vi "FPGA Main Default.vi"() -> ()   [LabVIEW 2019]
doc: "The myRIO v1.1 FPGA Shipping Personality. This personality contains support for:\n- 2 Analog Input Interrupt channel\n- 4 Digital Input Interrupt channel\n- 1 Timer\n- 1 Accelerometer\n- 1 Button\n- 4 LED\n- 10 Analog Input channels with 1 Sample\n- 6 Analog Output channels with 1 Sample\n- 40 Digital I/O channels with 1 Sample\n- 2 I2C channels\n- 4 Encoder channels\n- 6 PWM channels\n- 2 SPI channels"
uses:
  <vilib>/rvi/Emulation/niFpgaGetClockAttributes.vi
  <vilib>/rvi/Emulation/niFpgaSctlEmulationGetInTimedLoop.vi
  <vilib>/rvi/Emulation/niFpgaEmulationReportErrorSimple.vi
  <vilib>/rvi/Emulation/niFpgaProcessEmulError.vi
  <vilib>/rvi/eio/common/nirviEmuTemplateMethod_errors.vi
  <vilib>/rvi/Emulation/niFpgaCriticalErrorInLSC.vi
  <vilib>/eio/EIONode/EIONode.xnode
panel:
  in  "Synchronization":bool
  in  "OutputPinMap":u8
  out "PinMap":bool[](array[boolean])
  out "DIO_indicator":bool[](array[boolean])
  out "Camera_triggerin":bool
  out "Camera_triggerout":bool
  in  "PulseNumberperLoop":i32
  in  "Trigger":u64
  in  "BreakinLoop":bool
  in  "OFFTime":u32
  in  "ONTime":u32
  # "Camera trigger port: A:DIO8\nLight source port: B:DIO1~7, 1~6 are Normally Open (NO), 7 is  NC."
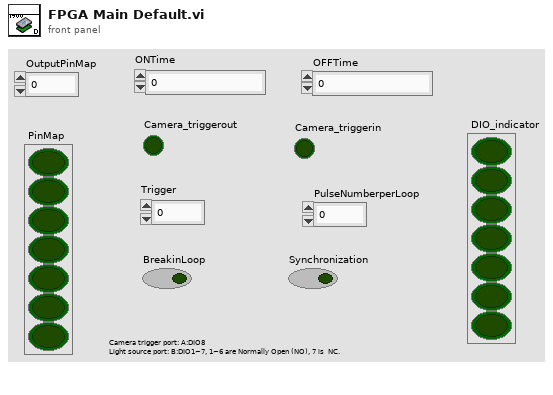
[diagram p1: front panel]
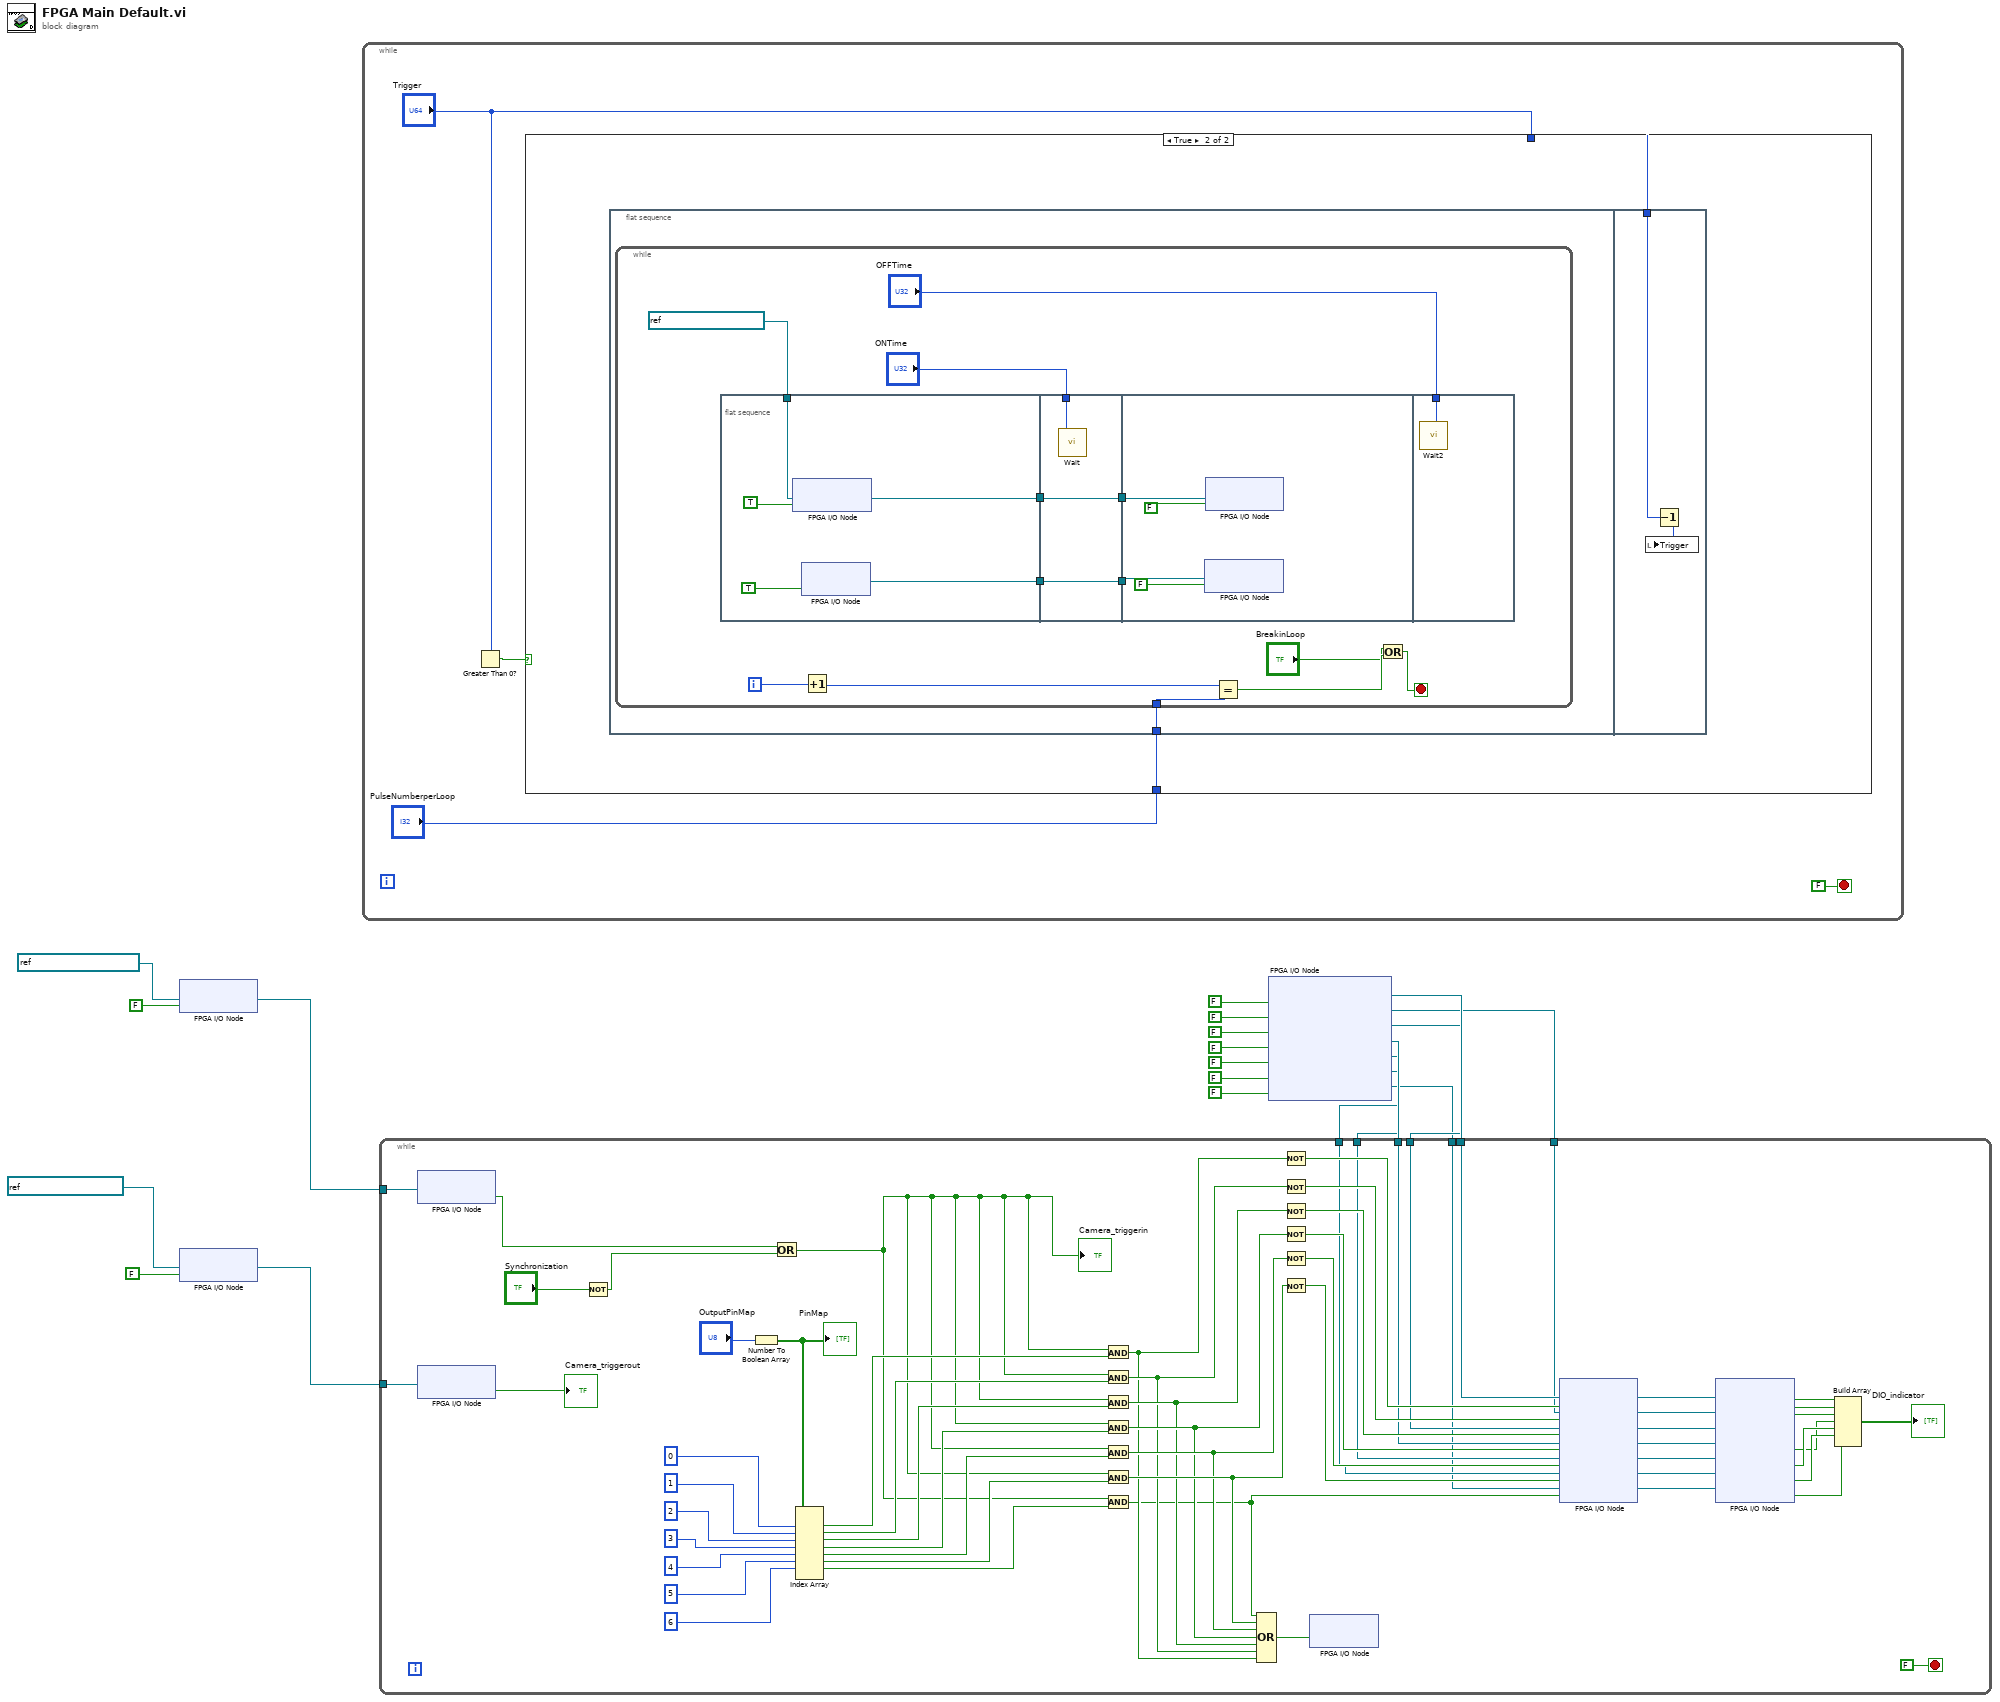
[diagram p0: block diagram]
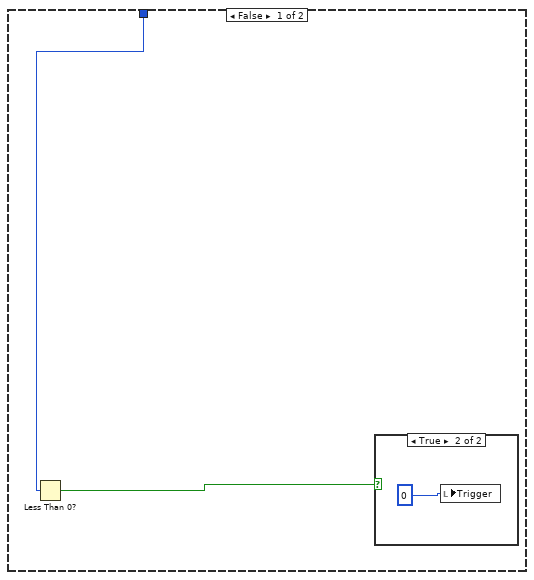
[diagram p2: hidden frame]
diagram:
  n1 = xnode "FPGA I/O Node"("I/O Item"=FALSE ("ConnectorB/DIO7"), "FPGA I/O In"=refnum<k21> "ConnectorA/DIO15") -> ("FPGA I/O Out"=w14:refnum<k21>)
  n2 = xnode "FPGA I/O Node"("I/O Item"=FALSE ("ConnectorA/DIO8"), "FPGA I/O In"=refnum<k21> "ConnectorA/DIO8") -> ("FPGA I/O Out"=w17:refnum<k21>)
  n3 = while {
    stop <- FALSE stop-if-true
    n4 = Greater Than 0?(x="Trigger") -> (x > 0?=w23:bool)
    n5 = case shown="True" w23 {
      tunnel: "PulseNumberperLoop" -> [_ w29]
      tunnel: "Trigger" -> [w26 w28]
      frame False {
        n6 = Less Than 0?(x=w26) -> (x < 0?=w25:bool)
        n7 = case shown="True" w25 {
          frame False {
          }
          frame True {
            n8 = local write "Trigger"(i16 0) -> ()
          }
        }
      }
      frame True {
        n9 = flat-sequence {
          tunnel: w29 -> [w30]
          tunnel: w28 -> [w57]
          frame #0 {
            n10 = while {
              tunnel: w30 -> [w38]
              i -> [w39]
              stop <- w41 stop-if-true
              n11 = flat-sequence {
                tunnel: refnum<k21> "ConnectorA/DIO8" ("FPGA I/O In") -> [w46]
                tunnel: [w45] -> w33
                tunnel: [w44] -> w31
                tunnel: "ONTime" -> [w51]
                tunnel: [w50] -> w34
                tunnel: w33 -> [w50]
                tunnel: [w49] -> w32
                tunnel: w31 -> [w49]
                tunnel: w34 -> [w53]
                tunnel: w32 -> [w52]
                tunnel: "OFFTime" -> [w56]
                frame #0 {
                  n12 = xnode "FPGA I/O Node"("I/O Item"=TRUE ("ConnectorA/DIO8"), "FPGA I/O In"=w46) -> ("FPGA I/O Out"=w44:refnum<k21>)
                  n13 = xnode "FPGA I/O Node"("LED0"=TRUE ("ConnectorA/DIO8")) -> ("FPGA I/O Out"=w45:refnum<k21>)  [unwired: 1 in]
                }
                frame #1 {
                  n14 = call "Wait"("Count(uSec)"=w51) -> ()  [unwired: 1 out]
                }
                frame #2 {
                  n15 = xnode "FPGA I/O Node"("I/O Item"=FALSE ("ConnectorA/DIO8"), "FPGA I/O In"=w53) -> ()  [unwired: 1 out]
                  n16 = xnode "FPGA I/O Node"("I/O Item"=FALSE ("ConnectorA/DIO8"), "FPGA I/O In"=w52) -> ()  [unwired: 1 out]
                }
                frame #3 {
                  n17 = call "Wait2"("Count(uSec)"=w56) -> ()  [unwired: 1 out]
                }
              }
              n18 = Increment(x=w39) -> (x+1=w40:i32)
              n19 = Equal?(x=w40, y=w38) -> (x = y?=w43:bool)
              n20 = Or(x="BreakinLoop", y=w43) -> (x .or. y?=w41:bool)
            }
          }
          frame #1 {
            n21 = Decrement(x=w57) -> (x-1=w58:u64)
            n22 = local write "Trigger"(w58) -> ()
          }
        }
      }
    }
  }
  n23 = xnode "FPGA I/O Node"("ConnectorB/DIO1"=FALSE ("ConnectorC/DIO1"), "ConnectorB/DIO2"=FALSE ("ConnectorC/DIO2"), "ConnectorB/DIO3"=FALSE ("ConnectorC/DIO3"), "ConnectorB/DIO4"=FALSE ("ConnectorC/DIO4"), "ConnectorB/DIO5"=FALSE ("ConnectorC/DIO5"), "ConnectorB/DIO6"=FALSE ("ConnectorC/DIO6"), "ConnectorB/DIO7"=FALSE ("ConnectorC/DIO7")) -> ("FPGA I/O Out"=w7:refnum<k21>, "FPGA I/O Out"=w6:refnum<k21>, "FPGA I/O Out"=w5:refnum<k21>, "FPGA I/O Out"=w4:refnum<k21>, "FPGA I/O Out"=w3:refnum<k21>, "FPGA I/O Out"=w2:refnum<k21>, "FPGA I/O Out"=w1:refnum<k21>)  [unwired: 7 in]
  n24 = while {
    tunnel: w17 -> [w71]
    tunnel: w14 -> [w70]
    tunnel: w7 -> [w69]
    tunnel: w6 -> [w68]
    tunnel: w5 -> [w67]
    tunnel: w4 -> [w66]
    tunnel: w3 -> [w65]
    tunnel: w2 -> [w64]
    tunnel: w1 -> [w63]
    stop <- FALSE stop-if-true
    n25 = xnode "FPGA I/O Node"("FPGA I/O In"=w70) -> ("I/O Item"=w59:bool)  [unwired: 1 out]
    n26 = xnode "FPGA I/O Node"("FPGA I/O In"=w71) -> ("I/O Item"=→"Camera_triggerout":bool)  [unwired: 1 out]
    n27 = Not(x="Synchronization") -> (.not. x?=w61:bool)
    n28 = Number To Boolean Array(number="OutputPinMap") -> (Boolean array=w99:bool[])
    "PinMap" <- w99
    n29 = Or(x=w59, y=w61) -> (x .or. y?=w60:bool)
    "Camera_triggerin" <- w60
    n30 = Index Array(array=w99, index #1=0 ("index"), index #2=1 ("index"), index #3=2 ("index"), index #4=3 ("index"), index #5=4 ("index"), index #6=5 ("index"), index #7=6 ("index")) -> (element #1=w106:bool, element #2=w105:bool, element #3=w104:bool, element #4=w103:bool, element #5=w102:bool, element #6=w101:bool, element #7=w100:bool)  [unwired: 1 in, 1 out]
    n31 = And(x=w60, y=w106) -> (x .and. y?=w93:bool)
    n32 = And(x=w60, y=w105) -> (x .and. y?=w94:bool)
    n33 = And(x=w60, y=w104) -> (x .and. y?=w95:bool)
    n34 = And(x=w60, y=w103) -> (x .and. y?=w96:bool)
    n35 = And(x=w60, y=w102) -> (x .and. y?=w97:bool)
    n36 = And(x=w60, y=w101) -> (x .and. y?=w98:bool)
    n37 = And(x=w60, y=w100) -> (x .and. y?=w87:bool)
    n38 = Compound Arithmetic op=OR(w87, w98, w97, w96, w95, w94, w93) -> (w92:bool)
    n39 = Not(x=w93) -> (.not. x?=w108:bool)
    n40 = Not(x=w94) -> (.not. x?=w109:bool)
    n41 = Not(x=w95) -> (.not. x?=w91:bool)
    n42 = Not(x=w96) -> (.not. x?=w90:bool)
    n43 = Not(x=w97) -> (.not. x?=w89:bool)
    n44 = Not(x=w98) -> (.not. x?=w88:bool)
    n45 = xnode "FPGA I/O Node"("LED1"=w92) -> ()  [unwired: 1 in, 1 out]
    n46 = xnode "FPGA I/O Node"("I/O Item"=w108, "FPGA I/O In"=w69, "I/O Item"=w109, "FPGA I/O In"=w68, "I/O Item"=w91, "FPGA I/O In"=w67, "I/O Item"=w90, "FPGA I/O In"=w66, "I/O Item"=w89, "FPGA I/O In"=w65, "I/O Item"=w88, "FPGA I/O In"=w64, "I/O Item"=w87, "FPGA I/O In"=w63) -> ("FPGA I/O Out"=w78:refnum<k21>, "FPGA I/O Out"=w77:refnum<k21>, "FPGA I/O Out"=w76:refnum<k21>, "FPGA I/O Out"=w75:refnum<k21>, "FPGA I/O Out"=w74:refnum<k21>, "FPGA I/O Out"=w73:refnum<k21>, "FPGA I/O Out"=w72:refnum<k21>)
    n47 = xnode "FPGA I/O Node"("FPGA I/O In"=w78, "FPGA I/O In"=w77, "FPGA I/O In"=w76, "FPGA I/O In"=w75, "FPGA I/O In"=w74, "FPGA I/O In"=w73, "FPGA I/O In"=w72) -> ("I/O Item"=w110:bool, "I/O Item"=w111:bool, "I/O Item"=w112:bool, "I/O Item"=w113:bool, "I/O Item"=w114:bool, "I/O Item"=w115:bool, "I/O Item"=w116:bool)  [unwired: 7 out]
    n48 = Build Array(w110, w111, w112, w113, w114, w115, w116) -> (→"DIO_indicator":bool[])
  }
